vi "Read Receive Binary Data queue.vi"(8 "error in (no error)":errorcluster, 11 "WebSocket Data Model in":refnum<class "WebSocket Data Model.lvclass">) -> (0 "error out":errorcluster, 2 "Receive Binary Data":refnum<queue>, 3 "WebSocket Data Model out":refnum<class "WebSocket Data Model.lvclass">)   [LabVIEW 2021, in "WebSockets.lvlib" / "WebSocket Data Model.lvclass"]
uses:
  WebSocket Data Model.lvclass
  WebSocket Data Model.lvclass/WebSocket Data Model.ctl
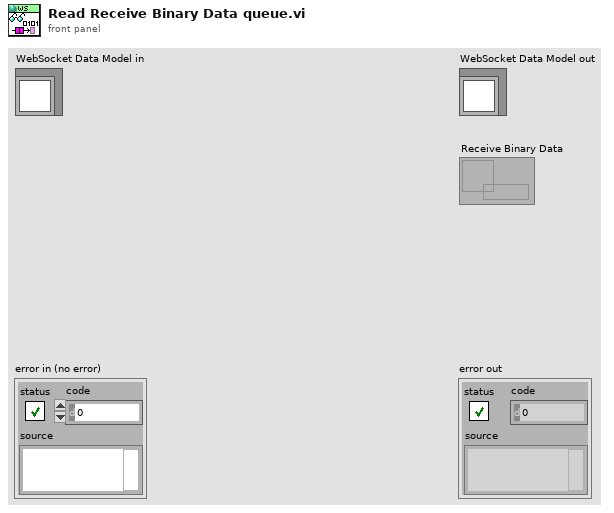
[diagram p1: front panel]
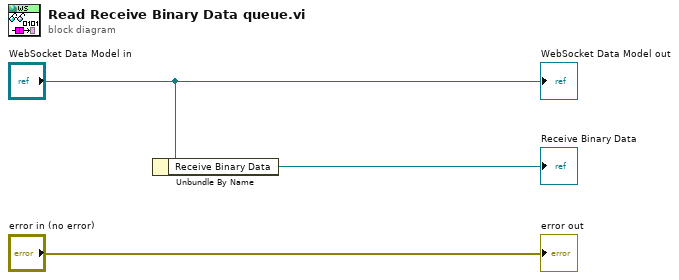
[diagram p0: block diagram]
diagram:
  n1 = Unbundle By Name("WebSocket Data Model in") -> ("Receive Binary Data"=→"Receive Binary Data":refnum<queue>)
  "error out" <- "error in (no error)"
  "WebSocket Data Model out" <- "WebSocket Data Model in"
